vi "CommonVIs SterotypeStringParser.vi"(0 "SterotypeStringIn":string) -> (12 "StereoType":T1=enum."APPLICATION", 14 "Name":string, 15 "SterotypeFound":bool, 16 "Sterotype":string)   [LabVIEW 2020]
uses:
  <resource>/Framework/Providers/Open_GDS/ClassProviders/Common/CommonVIs/CommonVIs_StereoType.ctl
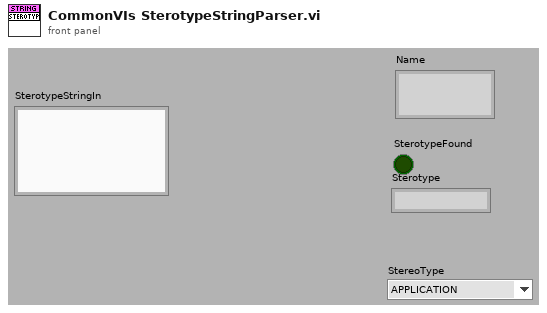
[diagram p1: front panel]
types:
  T1 = typedef "CommonVIs_StereoType.ctl" = enum16{"None", "TYPE", "ENUM", "ABSTRACT", "ACTOR", "GUI", "SINGLETON", "SIGNAL", "BOUNDARY", "ENTITY", "CONTROL", "LEGACY", "APPLICATION", "VI", "LVLIB", "INTERFACE"}
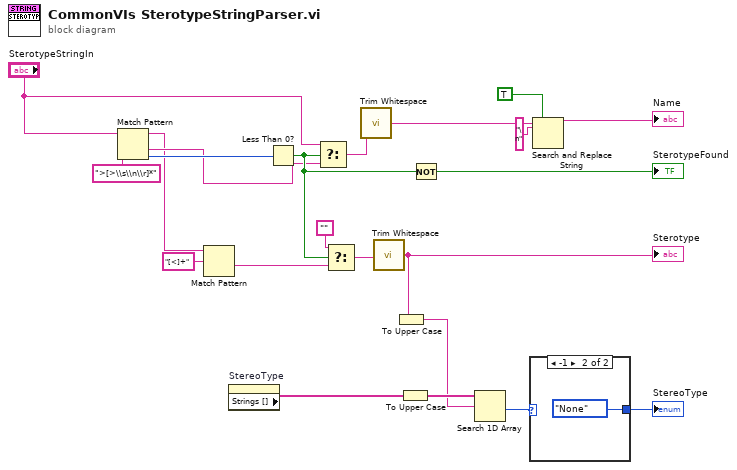
[diagram p0: block diagram]
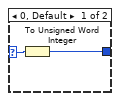
[diagram p2: hidden frame]
diagram:
  n1 = Match Pattern(string="SterotypeStringIn", regular expression=">[>\\s\\n\\r]*") -> (before substring=w14:string, after substring=w15:string, offset past match=w21:i32)  [unwired: 2 out]
  n2 = Match Pattern(string=w14, regular expression="[<]+") -> (after substring=w12:string)  [unwired: 4 out]
  n3 = property on="StereoType" class="Enum (strict)"() -> ("Strings []"=w10:string[])  [unwired: 2 in, 2 out]
  n4 = Less Than 0?(x=w21) -> (x < 0?=w17:bool)
  n5 = Select(t="SterotypeStringIn", s=w17, f=w15) -> (s? t:f=w19:string)
  n6 = Select(t="", s=w17, f=w12) -> (s? t:f=w11:string)
  n7 = call <vilib>:"Trim Whitespace.vi"("string"=w19) -> ("trimmed string"=w4:string)  [unwired: 1 in]
  n8 = call <vilib>:"Trim Whitespace.vi"("string"=w11) -> ("trimmed string"=w9:string)  [unwired: 1 in]
  "Sterotype" <- w9
  n9 = To Upper Case(1:w9) -> (0:w7:string)
  n10 = To Upper Case(1:w10) -> (0:w8:string[])
  n11 = Not(x=w17) -> (.not. x?=→"SterotypeFound":bool)
  n12 = Search 1D Array(1D array=w8, element=w7) -> (index of element=w5:i32)  [unwired: 1 out]
  n13 = case shown="-1" w5 {
    selector: w5 -> [w23 _]
    tunnel: [w24 CommonVIs_StereoType."None" ("StereoType")] -> w6
    frame 0, Default {
      n14 = To Unsigned Word Integer(number=w23) -> (unsigned 16bit integer=w24:u16)
    }
    frame -1 {
    }
  }
  "StereoType" <- w6
  n15 = Search and Replace String(replace all?=TRUE ("replace all? (F)"), input string=w4, search string="\n") -> (result string=→"Name":string)  [unwired: 1 in, 7 out]
